vi "PID Setpoint Profile Staged.vi"() -> ()   [LabVIEW 2019, in "control.lvlib"]
uses:
  control.lvlib
  Trigers/RS.vi
  Timer Delay/Timer.vi
  Inputs/Inputs.lvlib
  Userlib.lvlib
  Logik/Logik.lvlib
panel:
  out "Stop":bool
  out "Start 2":bool
  out "Elapsed time":dbl
  in  "Start":bool
  out "N curr":u32
  in  "t_tmp":u32[][](array[numeric])=[[0, 1], [0, 2], [0, 3], [0, 4], [0, 5], [0, 6], [0, 7], [0, 8], [0, 9], [0, 10], [0, 11], [0, 12], [0, 0], [0, 0], [0, 0], [0, 0], [0, 0], [0, 0], [0, 0], [0, 0], [0, 0]]
  out "t":u32
  out "profile complete?":bool
  in  "reinitialize? (F)":bool
  out "setpoint":dbl format="%.2f"
  in  "setpoint profile":cluster{"time (s)":dbl, "setpoint":dbl}[](array[cluster])=[{"time (s)"=0.0, "setpoint"=0.0}] {"setpoint" format="%.2f"; "time (s)" format="%.3f"}
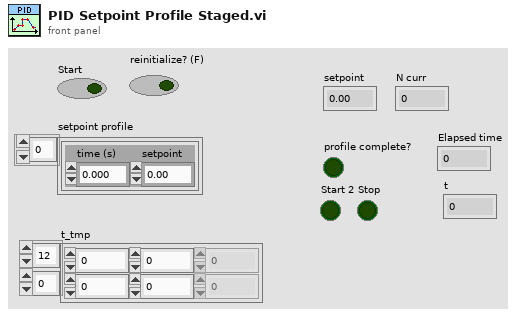
[diagram p1: front panel]
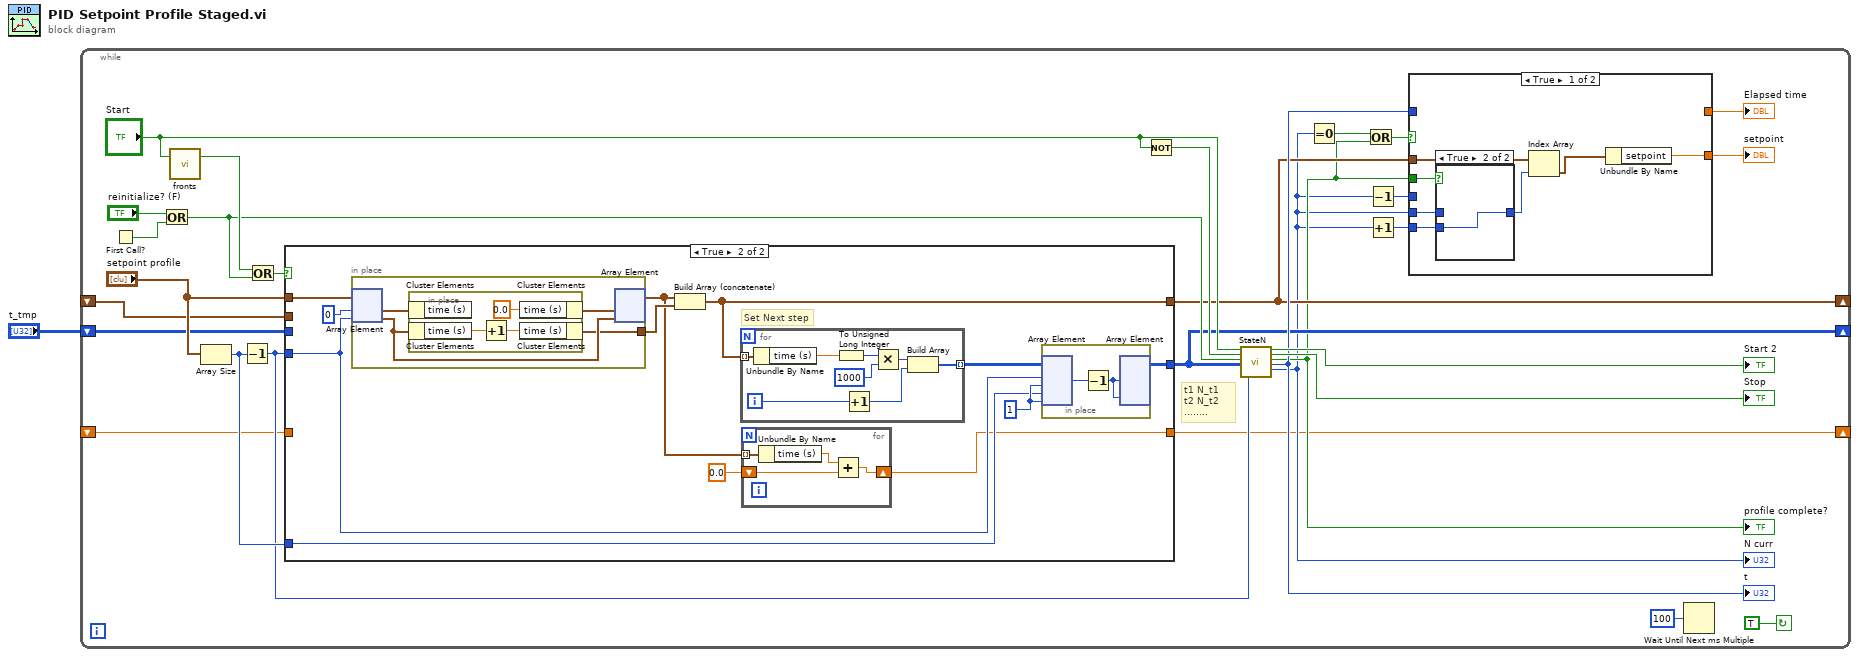
[diagram p0: block diagram]
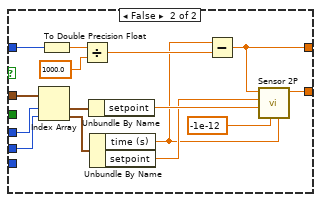
[diagram p4: hidden frame]
diagram:
  n1 = while {
    shift-right: [w16] -> _
    shift-left: "t_tmp" -> [w15]
    shift-right: [w14] -> _
    shift-left: _ -> [w13]
    shift-right: [w4] -> _
    shift-left: _ -> [w3]
    stop <- TRUE continue-if-true
    # "t1 N_t1\nt2 N_t2\n........"
    n2 = First Call?() -> (First Call?: T/F=w30:bool)
    n3 = Or(x="reinitialize? (F)", y=w30) -> (x .or. y?=w18:bool)
    n4 = call "fronts.vi"("in"="Start") -> ("raise"=w19:bool)  [unwired: 1 in, 1 out]
    n5 = Array Size(array="setpoint profile") -> (size(s)=w9:i32)
    n6 = Decrement(x=w9) -> (x-1=w5:i32)
    n7 = Or(x=w19, y=w18) -> (x .or. y?=w20:bool)
    n8 = case shown="True" w20 {
      tunnel: "setpoint profile" -> [_ w41]
      tunnel: [w33 w44] -> w16
      tunnel: w15 -> [w33 _]
      tunnel: w5 -> [_ w38]
      tunnel: [w32 w43] -> w14
      tunnel: w13 -> [w32 _]
      tunnel: w9 -> [_ w37]
      tunnel: [w31 w34] -> w4
      tunnel: w3 -> [w31 _]
      frame False {
      }
      frame True {
        w42 = 1
        # "Set Next step"
        n9 = in-place {
          in-place-border: [w50] -> w39
          n10 = in-place-array #1(w41, 0, w38) -> (w53:cluster{"time (s)":dbl, "setpoint":dbl}, w51:cluster{"time (s)":dbl, "setpoint":dbl})
          n11 = in-place {
            n12 = in-place-cluster #2(w53) -> ()  [unwired: 1 out]
            n13 = in-place-cluster #3(w51) -> ("time (s)"=w55:dbl)
            n14 = Increment(x=w55) -> (x+1=w54:dbl)
            n15 = in-place-cluster #2("time (s)"=0.0) -> (w52:cluster{"time (s)":dbl, "setpoint":dbl})
            n16 = in-place-cluster #3("time (s)"=w54) -> (w50:cluster{"time (s)":dbl, "setpoint":dbl})
          }
          n17 = in-place-array #1(w52, w51) -> (w36:cluster{"time (s)":dbl, "setpoint":dbl}[])  [unwired: 2 out]
        }
        n18 = Build Array (concatenate)(w36, w39) -> (w43:cluster{"time (s)":dbl, "setpoint":dbl}[])
        n19 = for {
          tunnel: w43 -> [w63] mode=indexing
          tunnel: [w61] -> w45 mode=indexing
          i -> [w60]
          n20 = Unbundle By Name(w63) -> ("time (s)"=w57:dbl)
          n21 = To Unsigned Long Integer(number=w57) -> (unsigned 32bit integer=w64:u32)
          n22 = Increment(x=w60) -> (x+1=w59:i32)
          n23 = Multiply(x=w64, y=u32 1000) -> (x*y=w62:u32)
          n24 = Build Array(w62, w59) -> (w61:u32[])
        }
        n25 = for {
          tunnel: w36 -> [w48] mode=indexing
          shift-right: [w47] -> w34
          shift-left: 0.0 -> [w46]
          n26 = Unbundle By Name(w48) -> ("time (s)"=w49:dbl)
          n27 = Add(x=w49, y=w46) -> (x+y=w47:dbl)
        }
        n28 = in-place {
          n29 = in-place-array #4(w45, w38, w42, w37, w42) -> (w66:u32)  [unwired: 1 out]
          n30 = Decrement(x=w66) -> (x-1=w65:u32)
          n31 = in-place-array #4(w65, w65) -> (w44:u32[][])  [unwired: 4 out]
        }
      }
    }
    n32 = Not(x="Start") -> (.not. x?=w27:bool)
    n33 = call "StateN.vi"("Start"="Start", "Stop"=w27, "Reset"=w18, "T_table"=w16, "End step"=w5) -> ("Start"=→"Start 2":bool, "Stop"=→"Stop":bool, "End"=w10:bool, "t"=w23:u32, "N curr"=w7:u32)  [unwired: 9 in, 1 out]
    "profile complete?" <- w10
    "t" <- w23
    "N curr" <- w7
    n34 = Equal To 0?(x=w7) -> (x = 0?=w11:bool)
    n35 = Or(x=w11, y=w10) -> (x .or. y?=w12:bool)
    n36 = Decrement(x=w7) -> (x-1=w8:u32)
    n37 = Increment(x=w7) -> (x+1=w6:u32)
    n38 = case shown="True" w12 {
      tunnel: w14 -> [w72 w88]
      tunnel: [w71 w87] -> w29
      tunnel: w8 -> [_ w86]
      tunnel: w23 -> [_ w83]
      tunnel: [_ w79] -> w22
      tunnel: w7 -> [w68 w82]
      tunnel: w10 -> [w70 _]
      tunnel: w6 -> [w67 _]
      frame True {
        n39 = case shown="True" w70 {
          tunnel: w68 -> [w74 _]
          tunnel: [w74 w75] -> w69
          tunnel: w67 -> [_ w75]
          frame False {
          }
          frame True {
          }
        }
        n40 = Index Array(array=w72, index=w69) -> (element=w73:cluster{"time (s)":dbl, "setpoint":dbl})
        n41 = Unbundle By Name(w73) -> ("setpoint"=w71:dbl)
      }
      frame False {
        n42 = Index Array(array=w88, index #1=w86, index #2=w82) -> (element #1=w90:cluster{"time (s)":dbl, "setpoint":dbl}, element #2=w89:cluster{"time (s)":dbl, "setpoint":dbl})
        n43 = To Double Precision Float(number=w83) -> (double precision float=w85:dbl)
        n44 = Divide(x=w85, y=1000.0) -> (x/y=w81:dbl)
        n45 = Unbundle By Name(w90) -> ("setpoint"=w78:dbl)
        n46 = Unbundle By Name(w89) -> ("time (s)"=w76:dbl, "setpoint"=w77:dbl)
        n47 = Subtract(x=w76, y=w81) -> (x-y=w79:dbl)
        n48 = call "Sensor 2P.vi"("Xmax"=w76, "Xmin"=-1e-12, "Ymin"=w78, "Ymax"=w77, "X"=w79) -> ("Y"=w87:dbl)  [unwired: 6 in]
      }
    }
    "setpoint" <- w29
    "Elapsed time" <- w22
    n49 = Wait Until Next ms Multiple(millisecond multiple=u32 100) -> ()  [unwired: 1 out]
  }
